vi "response_contentlength.vi"(11 "HTTP Request":T1) -> (3 "HTTP Request":T1)   [LabVIEW 2011]
uses:
  http_request_response.ctl
  http_request.ctl
  http_field.ctl
  http_response.ctl
  template_field.ctl
  template_field_type.ctl
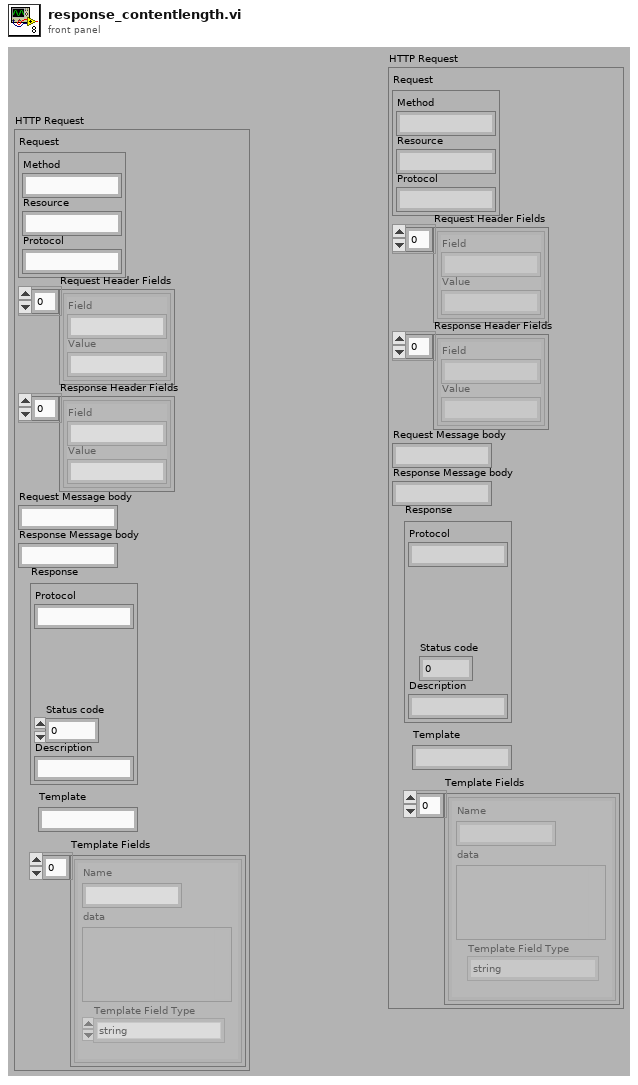
[diagram p1: front panel]
types:
  T1 = typedef "http_request_response.ctl" = cluster{"Request":T2, "Request Header Fields":T3[], "Response Header Fields":T3[], "Request Message body":string, "Response Message body":string, "Response":T4, "Template":string, "Template Fields":T5[]}
  T2 = typedef "http_request.ctl" = cluster{"Method":string, "Resource":string, "Protocol":string}
  T3 = typedef "http_field.ctl" = cluster{"Field":string, "Value":string}
  T4 = typedef "http_response.ctl" = cluster{"Protocol":string, "Status code":dbl, "Description":string}
  T5 = typedef "template_field.ctl" = cluster{"Name":string, "Template Field Type":T6, "data":variant}
  T6 = typedef "template_field_type.ctl" = enum16{"string", "string array", "number", "number array", "cluster", "cluster array"}
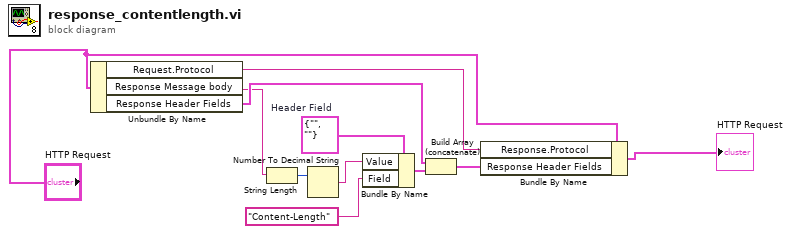
[diagram p0: block diagram]
diagram:
  w3 = T3 {"Field"="", "Value"=""}  # Header Field
  n1 = Unbundle By Name("HTTP Request") -> ("Request.Protocol"=w4:string, "Response Message body"=w9:string, "Response Header Fields"=w11:T3[])
  n2 = String Length(string=w9) -> (length=w7:i32)
  n3 = Number To Decimal String(number=w7) -> (decimal integer string=w8:string)  [unwired: 1 in]
  n4 = Bundle By Name(cluster=w3, "Value"=w8, "Field"="Content-Length") -> (w6:T3)
  n5 = Build Array (concatenate)(w11, w6) -> (w5:T3[])
  n6 = Bundle By Name(cluster="HTTP Request", "Response.Protocol"=w4, "Response Header Fields"=w5) -> (→"HTTP Request":T1)
